vi "Parameter.vi"(8 "error in (no error)":errorcluster, 11 "Node Ptr":T2 format="%.0x") -> (0 "error out":errorcluster)   [LabVIEW 2020, in "Ballard ARINC 429 System Explorer.lvlib" / "Implementation.lvlib"]
uses:
  Implementation.lvlib
  <vilib>/NI VeriStand/Custom Device API/Custom Device Item Ref.ctl
  Encoding and Decoding/Encoding.ctl
  <vilib>/NI VeriStand/Custom Device API/Custom Device API.lvlib
  Scripting/Ballard ARINC 429 Scripting.lvlib
  Encoding and Decoding/Encoding and Decoding.lvlib
panel:
  out "Unit":string
  out "Scale Offset":dbl
  out "Scale Factor":dbl=1.0
  out "Signed?":bool=TRUE
  out "Number of Bits":i32=10
  out "Start Bit":i32=18
  out "Default Value (Scaled)":dbl
  out "Encoding Type":T1
  in  "SHDocVw.IWebBrowser":refnum<k7>(container)
  in  "General Header":cluster{"Section Name":string}={"Section Name"="Ballard ARINC 429 - Parameter"}
  in  "Description":string
  out "Name":string
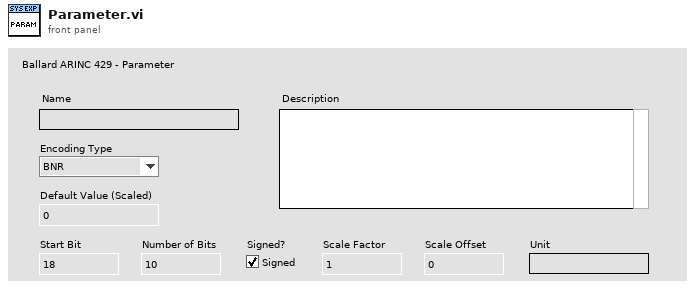
[diagram p1: front panel]
types:
  T1 = typedef "Encoding and Decoding.lvlib/Encoding.ctl" = enum16{"BNR", "BCD", "Discrete"}
  T2 = typedef "Custom Device API.lvlib/Custom Device Item Ref.ctl" = u64
  T3 = typedef "Custom Device API.lvlib/Custom Device Item Info.ctl" = cluster{"Name":string, "Is Channel":bool, "GUID":string, "Is Waveform":bool}
  T4 = typedef "Parameter Definition.ctl" = cluster{"start index":i32, "size":i32, "encoding":T1, "signed":bool, "scale multiplier":dbl, "scale offset":dbl}
  T5 = typedef "Custom Device API.lvlib/Custom Device Commands.ctl" = enum16{"Default", "Item renamed", "Shutdown", "Dynamic button pressed"}
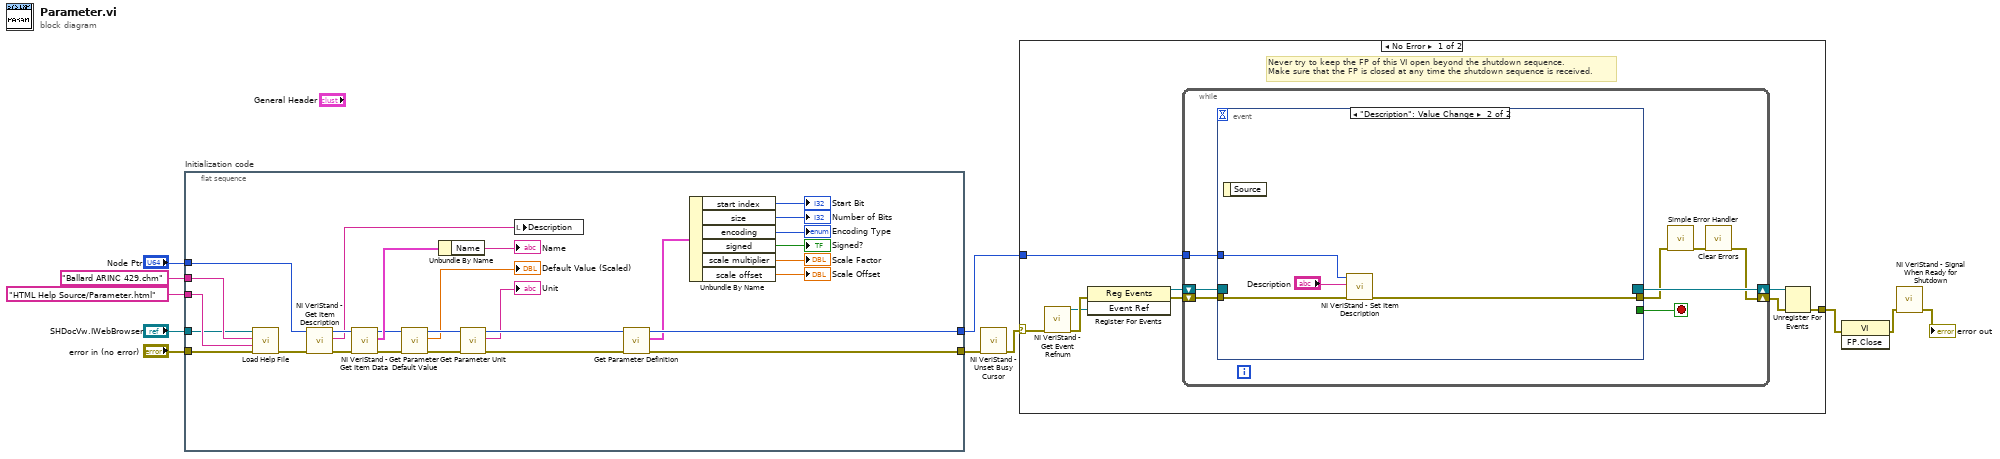
[diagram p0: block diagram]
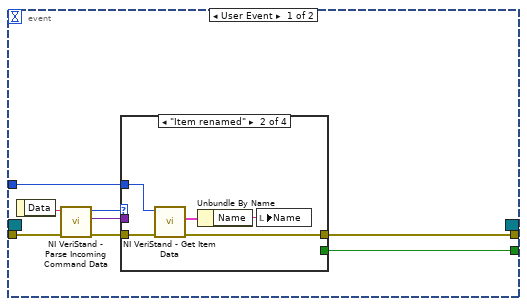
[diagram p2: hidden frame]
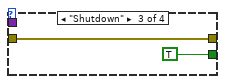
[diagram p4: hidden frame]
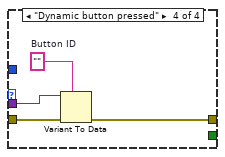
[diagram p5: hidden frame]
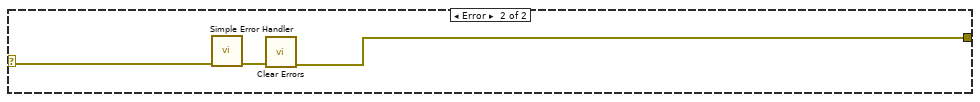
[diagram p6: hidden frame]
diagram:
  n1 = flat-sequence "Initialization code" {
    tunnel: "error in (no error)" -> [w34]
    tunnel: "Node Ptr" -> [w36]
    tunnel: [w28] -> w7
    tunnel: [w27] -> w4
    tunnel: "SHDocVw.IWebBrowser" -> [w30]
    tunnel: "HTML Help Source/Parameter.html" ("CD_CHM_Section") -> [w32]
    tunnel: "Ballard ARINC 429.chm" ("CD_CHM_FileName") -> [w31]
    frame #0 {
      n2 = call "Load Help File.vi"("error in (no error)"=w34, "HTML File to Load"=w32, "Main CHM File"=w31, "Browser"=w30) -> ("error out"=w33:errorcluster)  [unwired: 7 in]
      n3 = call <vilib>:"NI VeriStand - Get Item Description.vi"("error in (no error)"=w33, "Item Ref in"=w36) -> ("error out"=w38:errorcluster, "Description"=w35:string, "Item Ref out"=w39:T2)  [unwired: 7 out]
      n4 = call <vilib>:"NI VeriStand - Get Item Data.vi"("error in (no error)"=w38, "Item Ref in"=w39) -> ("error out"=w15:errorcluster, "Item Info"=w37:T3, "Item Ref out"=w16:T2)  [unwired: 7 out]
      n5 = call "Get Parameter Default Value.vi"("error in"=w15, "parameter ref"=w16) -> ("error out"=w14:errorcluster, "Default Value (Scaled)"=→"Default Value (Scaled)":dbl, "parameter ref out"=w13:T2)  [unwired: 7 in]
      n6 = Unbundle By Name(w37) -> ("Name"=→"Name":string)
      n7 = call "Get Parameter Unit.vi"("error in"=w14, "parameter ref"=w13) -> ("error out"=w19:errorcluster, "Unit"=→"Unit":string, "parameter ref out"=w18:T2)  [unwired: 7 in]
      n8 = local write "Description"(w35) -> ()
      n9 = call "Get Parameter Definition.vi"("error in"=w19, "parameter ref in"=w18) -> ("error out"=w28:errorcluster, "parameter definition"=w26:T4, "parameter ref out"=w27:T2)  [unwired: 7 in]
      n10 = Unbundle By Name(w26) -> ("start index"=→"Start Bit":i32, "size"=→"Number of Bits":i32, "encoding"=→"Encoding Type":T1, "signed"=→"Signed?":bool, "scale multiplier"=→"Scale Factor":dbl, "scale offset"=→"Scale Offset":dbl)
    }
  }
  n11 = call <vilib>:"NI VeriStand - Unset Busy Cursor.vi"("error in (no error)"=w7) -> ("error out"=w6:errorcluster)  [unwired: 10 out]
  n12 = case shown="No Error" w6 {
    selector: w6 -> [w40 w83]
    tunnel: [w45 w81] -> w11
    tunnel: w4 -> [w41 _]
    frame No Error {
      # "Never try to keep the FP of this VI open beyond the shutdown sequence.\nMake sure that the FP is closed at any time the shutdown sequence is received."
      n13 = call <vilib>:"NI VeriStand - Get Event Refnum.vi"("error in (no error)"=w40) -> ("error out"=w48:errorcluster, "Event Ref"=w44:refnum<user-event>)  [unwired: 9 out]
      n14 = register-events(error in=w48, w44) -> (reference out=w42:refnum<event-registration>, error out=w43:errorcluster)  [unwired: 1 in]
      n15 = while {
        tunnel: w41 -> [w52]
        shift-right: [w49] -> w46
        shift-left: w43 -> [w55]
        shift-right: [w56] -> w47
        shift-left: w42 -> [w54]
        stop <- w53 stop-if-true
        n16 = event shown="[1] \"Description\": Value Change" {
          selector: w54 -> [_ _]
          dyn-events: [_ _] -> w56
          timeout: _ -> [_ _]
          tunnel: w55 -> [w64 w79]
          tunnel: [w60 _] -> w53
          tunnel: [w59 w78] -> w51
          tunnel: w52 -> [w58 w80]
          event User Event {
            n17 = event-data() -> ("Data"=w63:string)  [unwired: 1 out]
            n18 = call <vilib>:"NI VeriStand - Parse Incoming Command Data.vi"("error in (no error)"=w64, "Incoming data"=w63) -> ("error out"=w62:errorcluster, "Outgoing data"=w57:variant, "Action"=w61:T5)  [unwired: 7 out]
            n19 = case shown="\"Item renamed\"" w61 {
              tunnel: w62 -> [w65 w70 w71 w76]
              tunnel: [_ _ TRUE _] -> w60
              tunnel: [w65 w67 w71 w73] -> w59
              tunnel: w58 -> [_ w69 _ _]
              tunnel: w57 -> [_ _ _ w75]
              frame "Default", Default {
              }
              frame "Item renamed" {
                n20 = call <vilib>:"NI VeriStand - Get Item Data.vi"("error in (no error)"=w70, "Item Ref in"=w69) -> ("error out"=w67:errorcluster, "Item Info"=w68:T3)  [unwired: 8 out]
                n21 = Unbundle By Name(w68) -> ("Name"=w66:string)
                n22 = local write "Name"(w66) -> ()
              }
              frame "Shutdown" {
              }
              frame "Dynamic button pressed" {
                w74 = ""  # Button ID
                n23 = Variant To Data(error in=w76, type=w74, Variant=w75) -> (error out=w73:errorcluster)  [unwired: 1 out]
              }
            }
          }
          event "Description": Value Change {
            n24 = event-data() -> ()  [unwired: 2 out]
            n25 = call <vilib>:"NI VeriStand - Set Item Description.vi"("error in (no error)"=w79, "Description"="Description", "Item Ref in"=w80) -> ("error out"=w78:errorcluster)  [unwired: 8 out]
          }
        }
        n26 = call <vilib>:"Simple Error Handler.vi"("error in (no error)"=w51) -> ("error out"=w50:errorcluster)  [unwired: 1 in, 7 out]
        n27 = call <vilib>:"Clear Errors.vi"("error in (no error)"=w50) -> ("error out"=w49:errorcluster)  [unwired: 1 in, 5 out]
      }
      n28 = Unregister For Events(event registration refnum=w47, error in=w46) -> (error out=w45:errorcluster)
    }
    frame Error {
      n29 = call <vilib>:"Simple Error Handler.vi"("error in (no error)"=w83) -> ("error out"=w82:errorcluster)  [unwired: 1 in, 7 out]
      n30 = call <vilib>:"Clear Errors.vi"("error in (no error)"=w82) -> ("error out"=w81:errorcluster)  [unwired: 1 in, 5 out]
    }
  }
  n31 = invoke class="VI" method="FP.Close"(error in=w11) -> (error out=w10:errorcluster)  [unwired: 2 in, 2 out]
  n32 = call <vilib>:"NI VeriStand - Signal When Ready for Shutdown.vi"("error in (no error)"=w10) -> ("error out"=→"error out":errorcluster)  [unwired: 10 out]
